vi "CSP_CalculateFilter.vi"(11 "CSP.lvclass":refnum<class "CSP.lvclass">) -> (3 "CSP.lvclass out":refnum<class "CSP.lvclass">)   [LabVIEW 2016, in "Spatial Pattern Filter.lvlib" / "CSP.lvclass"]
uses:
  CSP.lvclass
  CSP.lvclass/CSP.ctl
  <vilib>/Analysis/7linalg.llb/Complex Matrix Square Root.vi
  <vilib>/Analysis/baseanly.llb/Complex A x B.vi
  <vilib>/Analysis/7linalg.llb/Complex Eigenvalues and Vectors.vi
  <vilib>/Analysis/Matrix/Numeric/Add/Add - RM,RM.vi
  <vilib>/Analysis/7linalg.llb/Real Eigenvalues and Vectors.vi
  <vilib>/Analysis/7linalg.llb/Create Special Complex Matrix.vi
  <vilib>/Analysis/baseanly.llb/Complex Inverse Matrix.vi
  <vilib>/Analysis/Matrix/NI_Matrix.lvlib
  <vilib>/Analysis/NI_AALBase.lvlib
  <vilib>/Analysis/NI_AALPro.lvlib
  Spatial Pattern Filter.lvlib
panel:
  # "This VI is a part of BCI Design library, http://www.ru-bci.org \nCopyright © 2020, Sotnikov Peter, All rights reserved. License: GNU GPLv3"
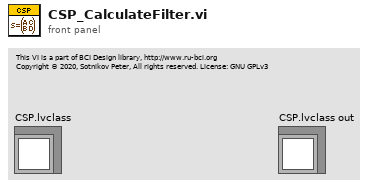
[diagram p1: front panel]
types:
  T1 = typedef "NI_Matrix.lvlib/RealMatrix.ctl" = dbl[][]
  T2 = cluster{"CSPMatrix":T1, "CovarianceMatrix1":T1, "CovarianceMatrix2":T1}[]
  T3 = typedef "NI_Matrix.lvlib/ComplexMatrix.ctl" = cdb[][]
  T4 = cluster{"CSPMatrix":T1, "CovarianceMatrix1":T1, "CovarianceMatrix2":T1}
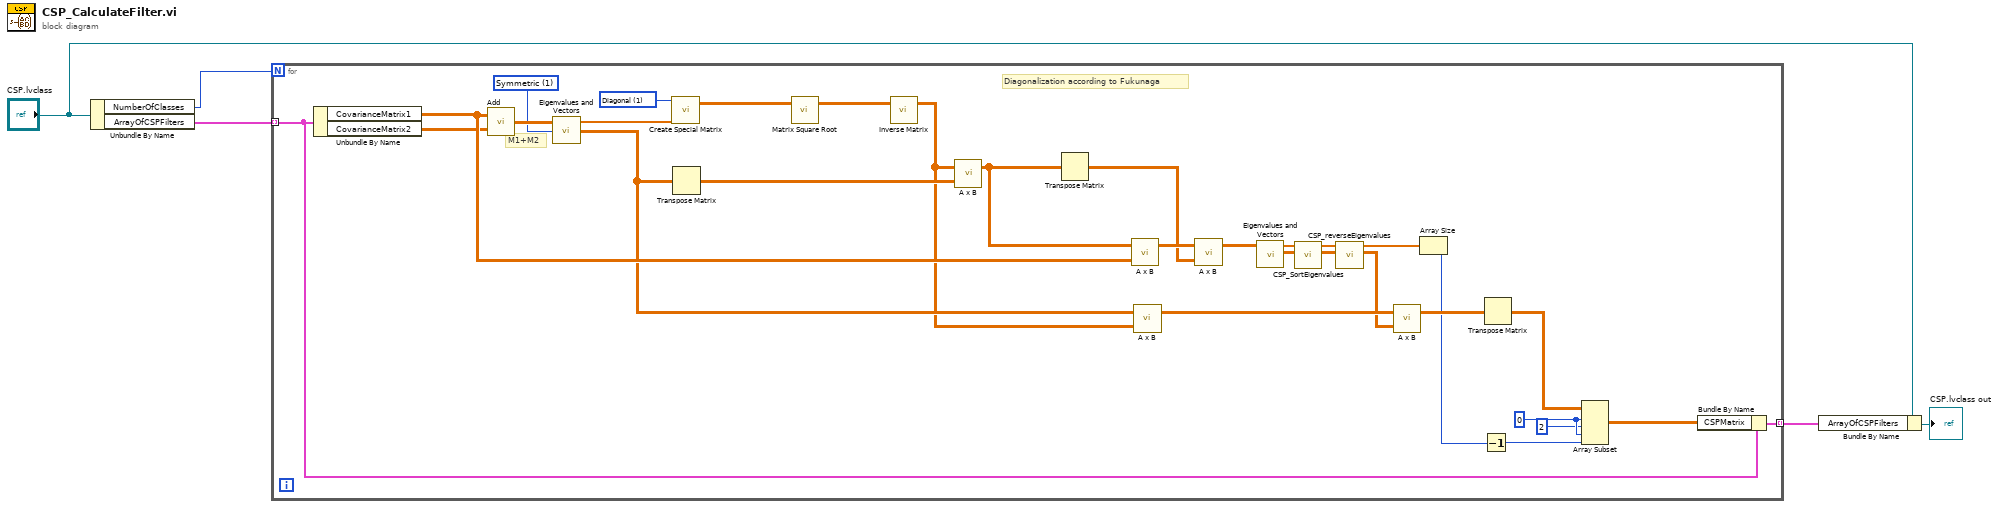
[diagram p0: block diagram]
diagram:
  n1 = Unbundle By Name("CSP.lvclass") -> ("NumberOfClasses"=w3:i32, "ArrayOfCSPFilters"=w5:T2)
  n2 = for {
    N: w3 -> [_]
    tunnel: w5 -> [w21] mode=indexing
    tunnel: [w36] -> w1 mode=indexing
    w12 = 0 ("row 1")
    w32 = 1 items=["Identity", "Diagonal", "Toeplitz", "Vandermonde", "Companion", "Hankel", "Hadamard", "Wilkinson", "Hilbert", "Inverse Hilbert", "Rosser", "Pascal"] ("matrix type")
    w34 = 1 items=["General", "Symmetric"] ("matrix type")
    # "M1+M2"
    # "Diagonalization according to Fukunaga"
    n3 = Unbundle By Name(w21) -> ("CovarianceMatrix1"=w27:T1, "CovarianceMatrix2"=w17:T1)
    n4 = call-poly <vilib>:"Add.vi"("Real Matrix B"=w17, "Real Matrix A"=w27) -> ("A + B"=w35:T1)
    n5 = call-poly <vilib>:"Eigenvalues and Vectors.vi"("matrix type"=w34, "Input Matrix"=w35) -> ("Eigenvectors"=w20:T3, "Eigenvalues"=w33:cdb[])  [unwired: 1 in, 1 out]
    n6 = call-poly <vilib>:"Create Special Matrix.vi"("matrix type"=w32, "Input Vector1"=w33) -> ("Special Matrix"=w31:T3)  [unwired: 3 in, 1 out]
    n7 = Transpose Matrix(1:w20) -> (0:w29:T3)
    n8 = call-poly <vilib>:"Matrix Square Root.vi"("Input Matrix"=w31) -> ("Matrix Square Root"=w30:T3)  [unwired: 1 in, 1 out]
    n9 = call-poly <vilib>:"Inverse Matrix.vi"("Input Matrix"=w30) -> ("Inverse Matrix"=w19:T3)  [unwired: 1 in, 1 out]
    n10 = call-poly <vilib>:"A x B.vi"("B"=w29, "A"=w19) -> ("A x B"=w28:T3)  [unwired: 1 out]
    n11 = Transpose Matrix(1:w28) -> (0:w25:T3)
    n12 = call-poly <vilib>:"A x B.vi"("B"=w27, "A"=w28) -> ("A x B"=w26:T3)  [unwired: 1 out]
    n13 = call-poly <vilib>:"A x B.vi"("B"=w19, "A"=w20) -> ("A x B"=w18:T3)  [unwired: 1 out]
    n14 = call-poly <vilib>:"A x B.vi"("B"=w25, "A"=w26) -> ("A x B"=w24:T3)  [unwired: 1 out]
    n15 = call-poly <vilib>:"Eigenvalues and Vectors.vi"("Input Matrix"=w24) -> ("Eigenvectors"=w22:T3, "Eigenvalues"=w23:cdb[])  [unwired: 2 in, 1 out]
    n16 = call "CSP_SortEigenvalues.vi"("Eigenvectors"=w22, "Eigenvalues"=w23) -> ("Eigenvectors Sorted"=w15:T3, "Eigenvalues Sorted"=w16:dbl[])  [unwired: 8 in]
    n17 = call "CSP_reverseEigenvalues.vi"("Eigenvectors in"=w15, "Eigenvalues in"=w16) -> ("Reversed Eigenvectors"=w14:T3, "Reversed Eigenvalues"=w9:cdb[])  [unwired: 6 in]
    n18 = call-poly <vilib>:"A x B.vi"("B"=w14, "A"=w18) -> ("A x B"=w8:T3)  [unwired: 1 out]
    n19 = Array Size(array=w9) -> (size(s)=w7:i32)
    n20 = Decrement(x=w7) -> (x-1=w6:i32)
    n21 = Transpose Matrix(1:w8) -> (0:w13:T3)
    n22 = Array Subset(array=w13, index (row)=w12, length (row)=2 ("row N"), index (col)=w12, length (col)=w6) -> (w11:T3)
    n23 = Bundle By Name(cluster=w21, "CSPMatrix"=w11) -> (w36:T4)
  }
  n24 = Bundle By Name(cluster="CSP.lvclass", "ArrayOfCSPFilters"=w1) -> (→"CSP.lvclass out":refnum<class "CSP.lvclass">)
